vi "Revision Query.vi"(8 "error in (no error)":errorcluster, 11 "VISA resource name":refnum<visa-resource-name>) -> (0 "error out":errorcluster, 1 "Instrument Firmware Revision":string, 2 "Instrument Driver Revision":string, 3 "VISA resource name out":refnum<visa-resource-name>)   [LabVIEW 2015, in "BK Precision 983X Series.lvlib"]
doc: "Queries the current instrument firmware revision and instrument driver revision.\n\nRefer to the Readme file for detailed driver information including modification history."
uses:
  <instrlib>/BK Precision 983X Series/BK Precision 983X Series.lvlib
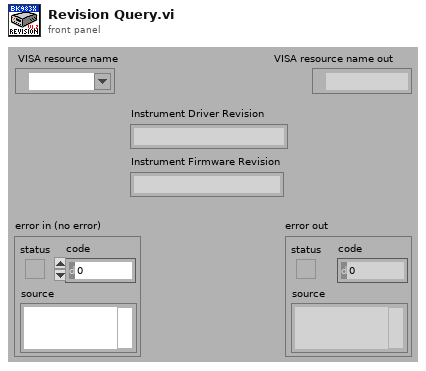
[diagram p1: front panel]
types:
  T1 = cluster{"Major":u16, "Minor":u16, "Fix":u16, "Build":u16}
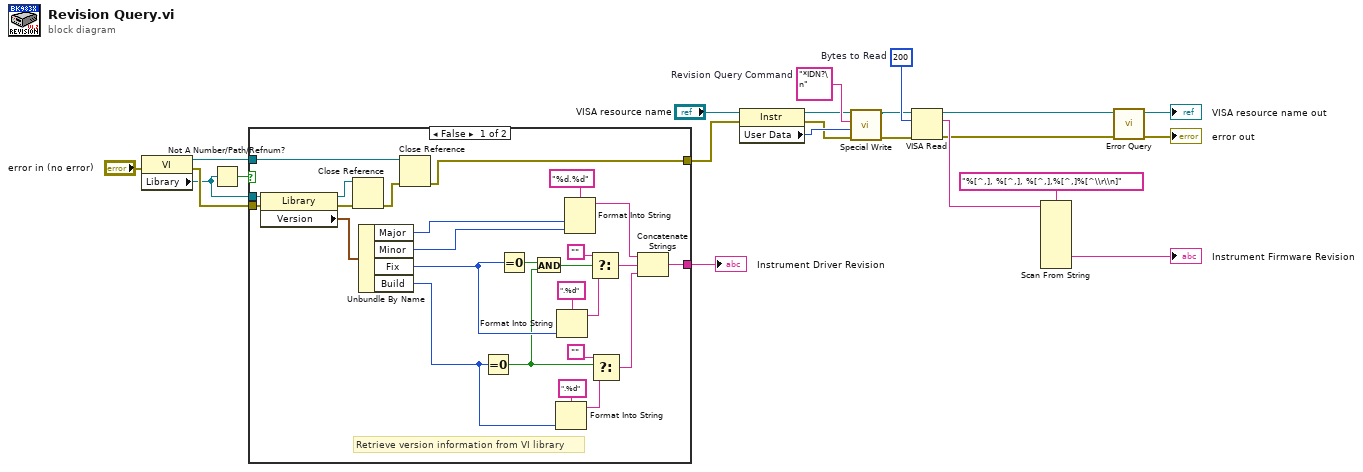
[diagram p0: block diagram]
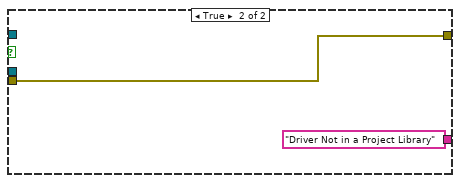
[diagram p2: hidden frame]
diagram:
  w10 = "*IDN?\n"  # Revision Query Command
  w21 = u32 200  # Bytes to Read
  n1 = property class="VI"(error in="error in (no error)") -> (reference out=w4:refnum<vi>, error out=w3:errorcluster, "Library"=w2:refnum<vi>)  [unwired: 1 in]
  n2 = Not A Number/Path/Refnum?(number/path/refnum=w2) -> (NaN/Path/Refnum?=w1:bool)
  n3 = case shown="False" w1 {
    tunnel: w4 -> [w45 _]
    tunnel: w3 -> [w30 w50]
    tunnel: [w25 w50] -> w8
    tunnel: [w24 "Driver Not in a Project Library"] -> w14
    tunnel: w2 -> [w23 _]
    frame False {
      # "Retrieve version information from VI library"
      n4 = property class="Library"(reference=w23, error in=w30) -> (reference out=w47:refnum<vi>, error out=w48:errorcluster, "Version"=w44:T1)
      n5 = Close Reference(reference=w47, error in (no error)=w48) -> (error out=w46:errorcluster)
      n6 = Unbundle By Name(w44) -> ("Major"=w33:u16, "Minor"=w32:u16, "Fix"=w29:u16, "Build"=w31:u16)
      n7 = Close Reference(reference=w45, error in (no error)=w46) -> (error out=w25:errorcluster)
      n8 = Equal To 0?(x=w31) -> (x = 0?=w27:bool)
      n9 = Equal To 0?(x=w29) -> (x = 0?=w28:bool)
      n10 = And(x=w28, y=w27) -> (x .and. y?=w26:bool)
      n11 = Format Into String(format string=".%d", w31) -> (resulting string=w37:string)  [unwired: 2 in, 1 out]
      n12 = Format Into String(format string=".%d", w29) -> (resulting string=w41:string)  [unwired: 2 in, 1 out]
      n13 = Format Into String(format string="%d.%d", w33, w32) -> (resulting string=w39:string)  [unwired: 2 in, 1 out]
      n14 = Select(t="", s=w26, f=w41) -> (s? t:f=w38:string)
      n15 = Select(t="", s=w27, f=w37) -> (s? t:f=w34:string)
      n16 = Concatenate Strings(w39, w38, w34) -> (w24:string)
    }
    frame True {
    }
  }
  "Instrument Driver Revision" <- w14
  n17 = property class="Instr"(reference="VISA resource name", error in=w8) -> (reference out=w5:refnum<visa-resource-name>, error out=w6:errorcluster, "User Data"=w7:u32)
  n18 = call <instrlib>:"Special Write.vi"("error in (no error)"=w6, "Delay (0 ms)"=w7, "Input String"=w10, "VISA resource name"=w5) -> ("error out"=w11:errorcluster, "VISA resource name out"=w12:refnum<visa-resource-name>)  [unwired: 6 in]
  n19 = VISA Read(VISA resource name=w12, byte count=w21, error in (no error)=w11) -> (VISA resource name out=w17:refnum<visa-resource-name>, read buffer=w20:string, error out=w18:errorcluster)  [unwired: 1 out]
  n20 = Scan From String(format string="%[^,], %[^,], %[^,],%[^,]%[^\\r\\n]", input string=w20) -> (output 4=→"Instrument Firmware Revision":string)  [unwired: 11 in, 3 out]
  n21 = call <instrlib>:"Error Query.vi"("error in (no error)"=w18, "VISA resource name"=w17) -> ("error out"=→"error out":errorcluster, "VISA resource name out"=→"VISA resource name out":refnum<visa-resource-name>)  [unwired: 6 in, 2 out]
